vi "OFBS_train_Mahalanobis.vi"(6 "Train Data":T1, 8 "error in (no error)":errorcluster, 10 "Parameters":i32[](array[numeric]), 11 "OFBS class in":refnum<class "OptFreqBandsSearch.lvclass">) -> (0 "error out":errorcluster, 1 "Mean vectors":dbl[][](array[numeric]), 2 "Covariance matricies (inversed)":dbl[][][](array[numeric]), 3 "OFBS class out":refnum<class "OptFreqBandsSearch.lvclass">)   [LabVIEW 2016, in "Optimal Frequency Bands Search.lvlib" / "OptFreqBandsSearch.lvclass"]
doc: "Метод, реализующий построение классификатора на основе многослойного персептрона. Для обучения классификатора используются обучающие данные."
uses:
  OptFreqBandsSearch.lvclass
  OFBS_DataTypes.ctl
  OptFreqBandsSearch.lvclass/OptFreqBandsSearch.ctl
  <vilib>/Analysis/baseanly.llb/Real Inverse Matrix.vi
  Optimal Frequency Bands Search.lvlib
  <vilib>/gmath/NI_Gmath.lvlib
  <vilib>/Analysis/NI_AALBase.lvlib
panel:
  out "Sizes":i32[](array[numeric])
  # "This VI is a part of BCI Design library, http://www.ru-bci.org \nCopyright © 2020, Sotnikov Peter, All rights reserved. License: GNU GPLv3"
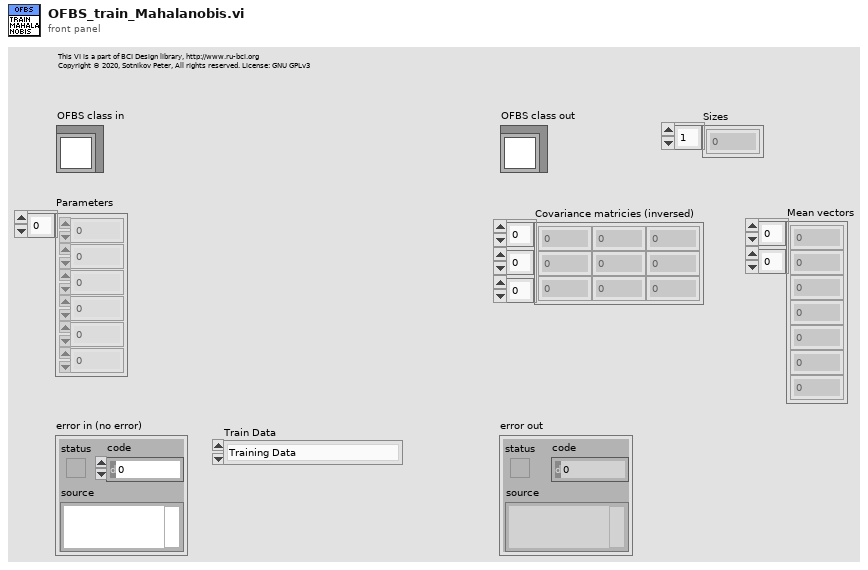
[diagram p1: front panel]
types:
  T1 = typedef "Optimal Frequency Bands Search.lvlib/OFBS_DataTypes.ctl" = enum16{"Training Data", "Test Data", "Training Data (cross-check)", "Test Data (cross-check)"}
  T2 = typedef "NI_Matrix.lvlib/RealMatrix.ctl" = dbl[][]
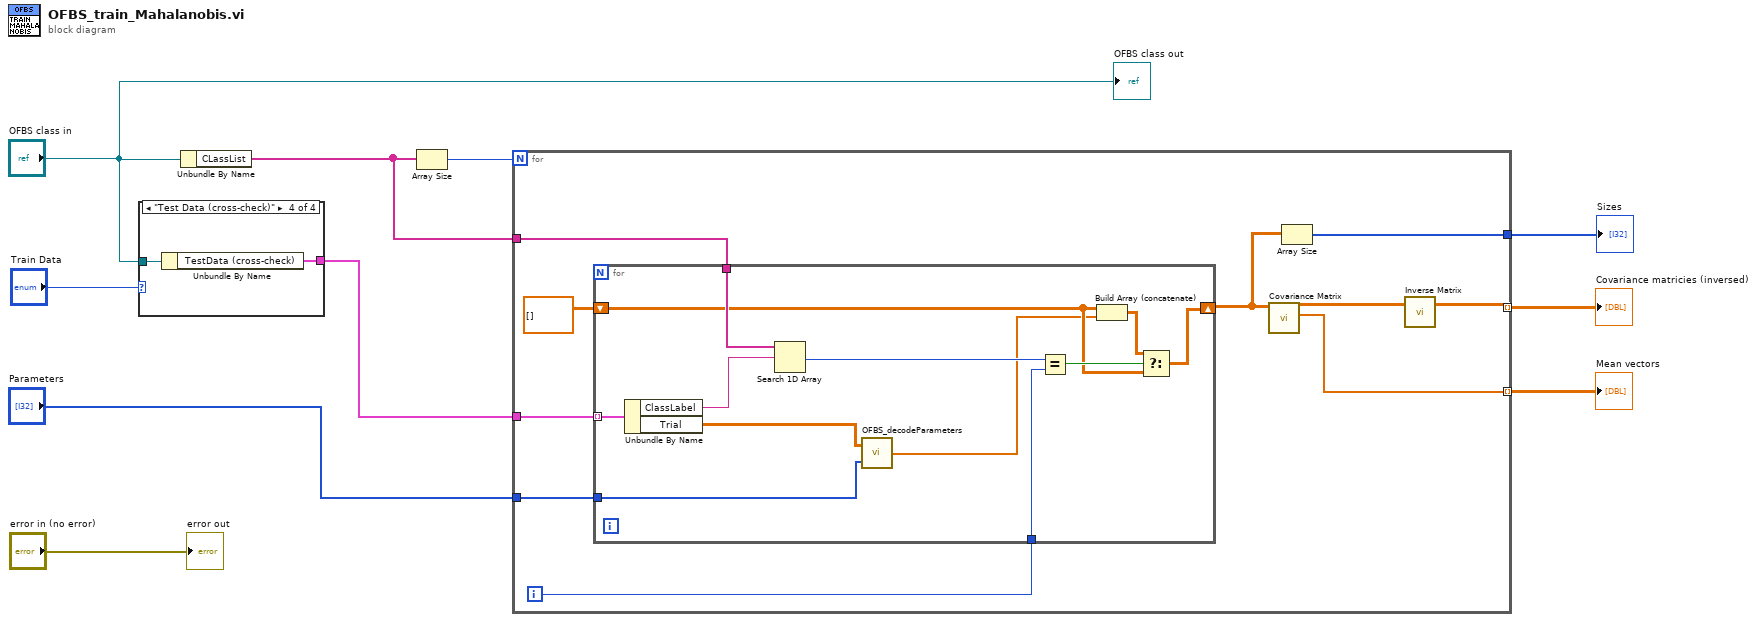
[diagram p0: block diagram]
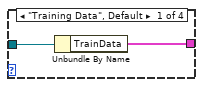
[diagram p2: hidden frame]
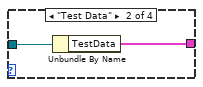
[diagram p3: hidden frame]
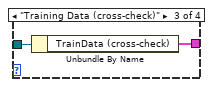
[diagram p4: hidden frame]
diagram:
  n1 = case shown="\"Test Data (cross-check)\"" "Train Data" {
    tunnel: "OFBS class in" -> [w12 w14 w16 w18]
    tunnel: [w11 w13 w15 w17] -> w2
    frame "Training Data", Default {
      n2 = Unbundle By Name(w12) -> ("TrainData"=w11:cluster{"ClassLabel":string, "Trial":dbl[][]}[])
    }
    frame "Test Data" {
      n3 = Unbundle By Name(w14) -> ("TestData"=w13:cluster{"ClassLabel":string, "Trial":dbl[][]}[])
    }
    frame "Training Data (cross-check)" {
      n4 = Unbundle By Name(w16) -> ("TrainData (cross-check)"=w15:cluster{"ClassLabel":string, "Trial":dbl[][]}[])
    }
    frame "Test Data (cross-check)" {
      n5 = Unbundle By Name(w18) -> ("TestData (cross-check)"=w17:cluster{"ClassLabel":string, "Trial":dbl[][]}[])
    }
  }
  n6 = Unbundle By Name("OFBS class in") -> ("CLassList"=w3:string[])
  n7 = Array Size(array=w3) -> (size(s)=w7:i32)
  n8 = for {
    N: w7 -> [_]
    tunnel: "Parameters" -> [w28]
    tunnel: w2 -> [w27]
    tunnel: w3 -> [w26]
    tunnel: [w19] -> w5 mode=indexing
    tunnel: [w23] -> w4 mode=indexing
    tunnel: [w21] -> w6
    i -> [w25]
    n9 = for {
      tunnel: w27 -> [w40] mode=indexing
      tunnel: w28 -> [w30]
      tunnel: w26 -> [w39]
      tunnel: w25 -> [w36]
      shift-right: [w32] -> w22
      shift-left: dbl[][] [] -> [w33]
      n10 = Unbundle By Name(w40) -> ("ClassLabel"=w38:string, "Trial"=w31:dbl[][])
      n11 = Search 1D Array(1D array=w39, element=w38) -> (index of element=w37:i32)  [unwired: 1 in]
      n12 = call "OFBS_decodeParameters.vi"("Parameters"=w30, "Trial"=w31) -> ("FeatureVector"=w29:dbl[])
      n13 = Equal?(x=w37, y=w36) -> (x = y?=w35:bool)
      n14 = Build Array (concatenate)(w33, w29) -> (w34:dbl[][])
      n15 = Select(t=w34, s=w35, f=w33) -> (s? t:f=w32:dbl[][])
    }
    n16 = call <vilib>:"Covariance Matrix.vi"("X"=w22) -> ("mean vector"=w23:dbl[], "covariance matrix V"=w20:T2)  [unwired: 9 in]
    n17 = Array Size(array=w22) -> (size(s)=w21:i32[])
    n18 = call-poly <vilib>:"Inverse Matrix.vi"("Input Matrix"=w20) -> ("Inverse Matrix"=w19:T2)  [unwired: 1 in, 1 out]
  }
  "Sizes" <- w6
  "Covariance matricies (inversed)" <- w5
  "Mean vectors" <- w4
  "error out" <- "error in (no error)"
  "OFBS class out" <- "OFBS class in"
